vi "Destroy User Events.vi"(8 "error in (no error)":errorcluster, 11 "User Event in":refnum<class "User Event.lvclass">) -> (0 "error out":errorcluster, 3 "User Event out":refnum<class "User Event.lvclass">)   [LabVIEW 2016, in "User Event.lvclass"]
uses:
  User Event.lvclass
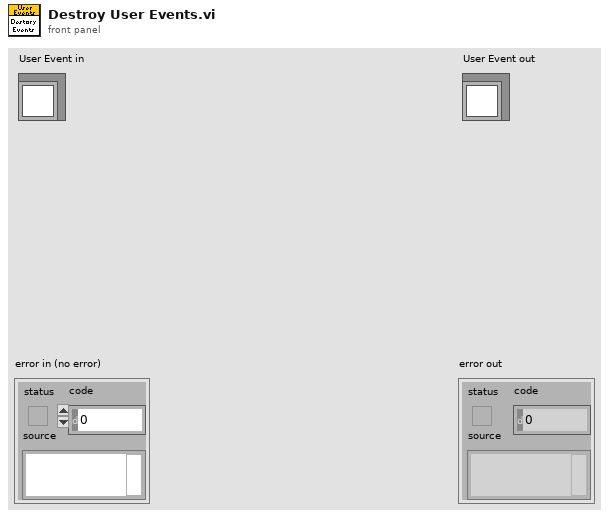
[diagram p1: front panel]
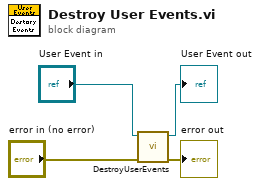
[diagram p0: block diagram]
diagram:
  n1 = call "DestroyUserEvents.vi"("error in (no error)"="error in (no error)", "User Event in"="User Event in") -> ("error out"=→"error out":errorcluster, "User Event out"=→"User Event out":refnum<class "User Event.lvclass">)  [unwired: 8 in]
